vi "test_Find Local Chassis Returns Modules.vi"(8 "error in (no error)":errorcluster, 11 "TestCase in":refnum<class "Scan Engine Scripting API Custom Device Unit Tests.lvclass">) -> (0 "error out":errorcluster, 3 "TestCase out":refnum<class "Scan Engine Scripting API Custom Device Unit Tests.lvclass">)   [LabVIEW 2017, in "Scan Engine Scripting API Custom Device Unit Tests.lvclass"]
uses:
  Scan Engine Scripting API Custom Device Unit Tests.lvclass
  Type Defs/Local Chassis Settings.ctl
  Scan Engine Scripting API Custom Device Unit Tests.lvclass/Scan Engine Scripting API Custom Device Unit Tests.ctl
  Type Defs/Main Settings.ctl
  <vilib>/addons/_JKI Toolkits/VI Tester/TestCase.llb/TestCase.lvclass
  Scripting/Scan Engine Scripting.lvlib
  Scan Engine Custom Device.lvlib
  C:/Program Files (x86)/National Instruments/LabVIEW 2017/vi.lib/addons/_JKI Toolkits/VI Tester/TestCase.llb/TestCase.lvclass
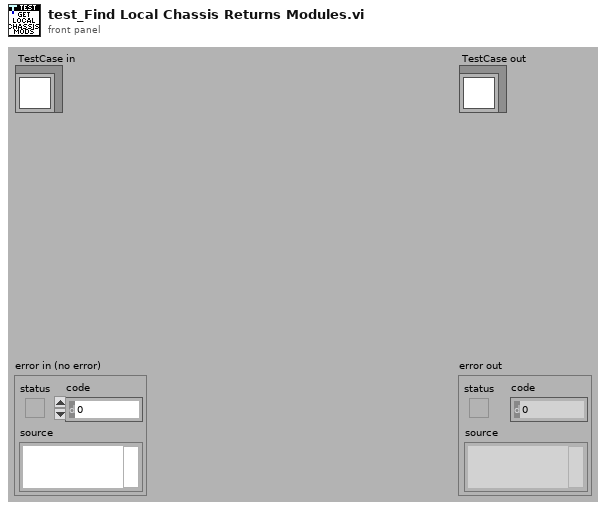
[diagram p1: front panel]
types:
  T1 = typedef "Scan Engine Custom Device.lvlib/Local Chassis Settings.ctl" = cluster{"name":string, "number of slots":i32}
  T2 = typedef "Scan Engine Custom Device.lvlib/Main Settings.ctl" = cluster{"sync to scan":bool, "scan engine decimation":u16, "delay after FPGA load (s)":u16}
  T3 = typedef "Custom Device API.lvlib/Custom Device Item Ref.ctl" = u64
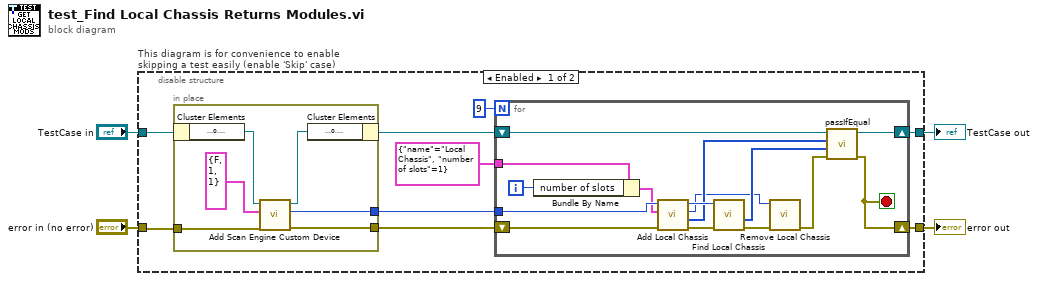
[diagram p0: block diagram]
diagram:
  n1 = disable-structure "This diagram is for convenience to enable skipping a test easily (enable 'Skip' case)" shown="Enabled" {
    disable-tunnel: "TestCase in" -> [w7 w38]
    disable-tunnel: [w8 w36] -> w1
    disable-tunnel: [w13 w37] -> w3
    disable-tunnel: "error in (no error)" -> [w9 w35]
    frame Enabled {
      n2 = in-place {
        in-place-border: [w34] -> w11
        in-place-border: [w33] -> w10
        in-place-border: w9 -> [w31]
        n3 = in-place-cluster #1(w7) -> ("target ref"=w30:refnum<k24>)
        n4 = call "Add Scan Engine Custom Device.vi"("error in"=w31, "settings"=T2 {"sync to scan"=FALSE, "scan engine decimation"=1, "delay after FPGA load (s)"=1}, "target in"=w30) -> ("error out"=w33:errorcluster, "scan engine custom device ref"=w34:T3, "target out"=w29:refnum<k24>)  [unwired: 6 in]
        n5 = in-place-cluster #1("target ref"=w29) -> (w6:refnum<class "Scan Engine Scripting API Custom Device Unit Tests.lvclass">)
      }
      n6 = for {
        N: 9 -> [_]
        tunnel: T1 {"name"="Local Chassis", "number of slots"=1} ("settings") -> [w28]
        tunnel: w11 -> [w27]
        shift-right: [w14] -> w13
        shift-left: w10 -> [w26]
        shift-right: [w22] -> w8
        shift-left: w6 -> [w23]
        i -> [w17]
        stop <- w14 stop-if-true
        n7 = Bundle By Name(cluster=w28, "number of slots"=w17) -> (w18:T1)
        n8 = call "Add Local Chassis.vi"("error in"=w26, "settings"=w18, "scan engine custom device ref in"=w27) -> ("error out"=w24:errorcluster, "slot refs"=w20:T3[], "local chassis ref"=w15:T3, "scan engine custom device ref out"=w25:T3)  [unwired: 4 in, 1 out]
        n9 = call "Find Local Chassis.vi"("error in"=w24, "scan engine custom device ref in"=w25) -> ("error out"=w21:errorcluster, "slots refs"=w19:T3[])  [unwired: 5 in, 3 out]
        n10 = call "Remove Local Chassis.vi"("error in"=w21, "local chassis ref"=w15) -> ("error out"=w16:errorcluster)  [unwired: 9 in]
        n11 = call-dynamic "passIfEqual.vi"("error in (no error)"=w16, "y"=w19, "x"=w20, "TestCase in"=w23) -> ("error out"=w14:errorcluster, "TestCase out"=w22:refnum<class "Scan Engine Scripting API Custom Device Unit Tests.lvclass">)  [unwired: 6 in]
      }
    }
    frame Disabled {
      # "skip test result while test is under development"
      n12 = call <vilib>:"skip.vi"("error in (no error)"=w35, "TestCase in"=w38) -> ("error out"=w37:errorcluster, "TestCase out"=w36:refnum<class "Scan Engine Scripting API Custom Device Unit Tests.lvclass">)  [unwired: 8 in]
    }
  }
  "error out" <- w3
  "TestCase out" <- w1
